vi "Config.vi"(8 "error in (no error)":errorcluster, 10 "Setting":variant, 11 "niPower in":refnum<class "NI DC Power.lvclass">) -> (0 "error out":errorcluster, 3 "niPower out":refnum<class "NI DC Power.lvclass">)   [LabVIEW 2025, in "Power Supply.lvlib" / "NI DC Power.lvclass"]
uses:
  NI DC Power.lvclass
  <instrlib>/niDCPower/nidcpower.llb/niDCPower Wait For Event - Event.ctl
  PS Channel/Power Supply Channel.lvclass
  NI DC Power.lvclass/NI DC Power.ctl
  <instrlib>/niDCPower/nidcpower.llb/niDCPower Output Function.ctl
  <instrlib>/niDCPower/nidcpower.llb/niDCPower Source Mode.ctl
  Users/Public/Documents/Sandia National Labs/TSS Plugin/Abstract Engine.lvlibp/Plugin/Abstract/Abstract Instrument/Channel.ctl
  PS Channel configuration/Power Supply Channel configuration.lvclass
  PS Channel configuration/Power Supply Channel configuration.lvclass/Power Supply Channel configuration.ctl
  PS Channel configuration/Read PS Channel.vi
  Users/Public/Documents/Sandia National Labs/TSS Plugin/CEF.lvlibp/Node/ReadChildren.vi
  Users/Public/Documents/Sandia National Labs/TSS Plugin/Abstract Engine.lvlibp/Plugin/Abstract/Channel configuration/Read Channel Setting.vi
  Users/Public/Documents/Sandia National Labs/TSS Plugin/CEF.lvlibp/Node/CEF_Node.lvclass
  Users/Public/Documents/Sandia National Labs/TSS Plugin/CEF.lvlibp/serializable configuration/CEF_serializable configuration.lvclass
  Users/Public/Documents/Sandia National Labs/TSS Plugin/Abstract Engine.lvlibp/Plugin/Abstract/Abstract Instrument/Abstract Instrument.lvclass
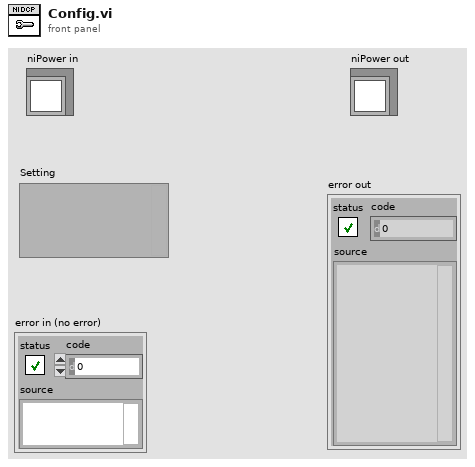
[diagram p1: front panel]
types:
  T1 = typedef "niDCPower Wait For Event - Event.ctl" = i32
  T2 = typedef "Abstract Engine.lvlibp/Abstract Instrument.lvclass/Channel.ctl" = cluster{"Alias":string, "DataType":enum16{"Anaolg Input", "Waveform"}, "Unit":enum16{"---", "V", "A", "Ohm", "Hz", "uF", "degC", "deg"}, "Upper limit":dbl, "Lower limit":dbl, "Measurement":variant}
  T3 = typedef "niDCPower Source Mode.ctl" = i32
  T4 = typedef "niDCPower Output Function.ctl" = i32
  T5 = typedef "Power Supply.lvlib/Power Supply Channel configuration.lvclass/PS Channel Setting.ctl" = cluster{"Driver":string, "Pin":string, "Test Voltage":string, "Voltage Low":dbl, "Voltage Norminal":dbl, "Voltage High":dbl, "PreTest Voltage":dbl, "PreTest Current":dbl, "Current Limit":dbl}
  T6 = typedef "Abstract Engine.lvlibp/Channel configuration.lvclass/Default Channel.ctl" = cluster{"Address":string, "SW Alias":string, "Enabled":bool, "Type":string, "Description":string}
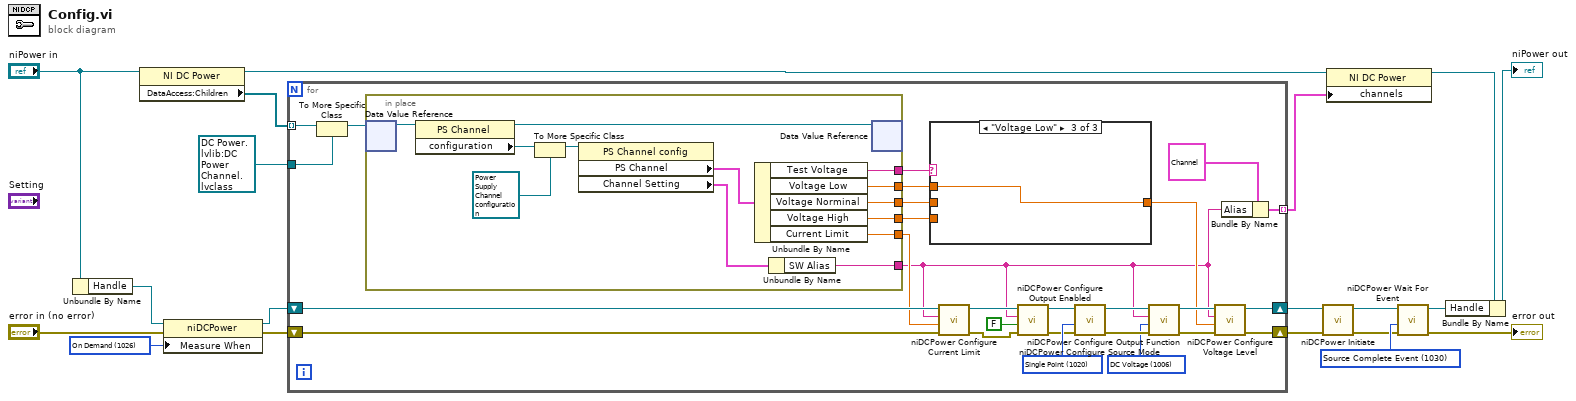
[diagram p0: block diagram]
diagram:
  w9 = 1026 items=["Automatically after Source Complete"=1025, "On Demand"=1026, "On Measure Trigger"=1027] ("Measurement:Advanced:Measure When")
  w17 = T1 1030 items=["Source Complete Event"=1030, "Measure Complete Event"=1031, "Sequence Iteration Complete Event"=1032, "Sequence Engine Done Event"=1033, "Pulse Complete Event"=1051, "Ready For Pulse Trigger Event"=1052] ("event")
  n1 = Unbundle By Name("niPower in") -> ("Handle"=w6:refnum<k15>)
  n2 = property class="NI DC Power"(reference="niPower in") -> (reference out=w12:refnum<class "NI DC Power.lvclass">, "DataAccess:Children"=w11:refnum<data-value>[])  [unwired: 1 in, 1 out]
  n3 = property class="niDCPower"(reference=w6, error in="error in (no error)", "Measure When"=w9) -> (reference out=w5:refnum<k15>, error out=w7:errorcluster)
  n4 = for {
    shift-right: [w27] -> w3
    shift-left: w5 -> [w26]
    shift-right: [w28] -> w4
    shift-left: w7 -> [w25]
    tunnel: w11 -> [w37] mode=indexing
    tunnel: refnum<data-value> refnum ("data value reference") -> [w35]
    tunnel: [w34] -> w1 mode=indexing
    w41 = T3 1020 items=["Single Point"=1020, "Sequence"=1021] ("source mode")
    w42 = T4 1006 items=["DC Voltage"=1006, "DC Current"=1007, "Pulse Voltage"=1049, "Pulse Current"=1050] ("output function")
    n5 = To More Specific Class(target class=w35, reference=w37) -> (specific class reference=w36:refnum<data-value>)  [unwired: 1 in, 1 out]
    n6 = in-place {
      in-place-border: [w47] -> w22
      in-place-border: [w57] -> w21
      in-place-border: [w51] -> w33
      in-place-border: [w50] -> w32
      in-place-border: [w49] -> w31
      in-place-border: [w48] -> w30
      # "Initialize the front panel controls when loaded"
      n7 = in-place-dvr #1(w36) -> (w59:refnum<class "Power Supply Channel.lvclass">)  [unwired: 1 out]
      n8 = property class="PS Channel"(reference=w59) -> (reference out=w58:refnum<class "Power Supply Channel.lvclass">, "configuration"=w56:refnum<class "CEF_serializable configuration.lvclass">)  [unwired: 1 in, 1 out]
      n9 = To More Specific Class(target class=refnum<class "Power Supply Channel configuration.lvclass"> refnum ("DC Power.lvlib:DCPower Channel configuration.lvclass"), reference=w56) -> (specific class reference=w55:refnum<class "Power Supply Channel configuration.lvclass">)  [unwired: 1 in, 1 out]
      n10 = property class="PS Channel config"(reference=w55) -> ("PS Channel"=w53:T5, "Channel Setting"=w52:T6)  [unwired: 1 in, 2 out]
      n11 = Unbundle By Name(w53) -> ("Test Voltage"=w51:string, "Voltage Low"=w50:dbl, "Voltage Norminal"=w49:dbl, "Voltage High"=w48:dbl, "Current Limit"=w47:dbl)
      n12 = Unbundle By Name(w52) -> ("SW Alias"=w57:string)
      n13 = in-place-dvr #1(w58) -> ()  [unwired: 2 out]
    }
    n14 = case shown="\"Voltage Low\"" w33 {
      tunnel: w32 -> [_ _ w62]
      tunnel: w31 -> [w60 _ _]
      tunnel: w30 -> [_ w61 _]
      tunnel: [w60 w61 w62] -> w29
      frame "Voltage Norminal", Default {
      }
      frame "Voltage High" {
      }
      frame "Voltage Low" {
      }
    }
    n15 = call <instrlib>:"niDCPower Configure Current Limit.vi"("error in (no error)"=w25, "current limit"=w22, "channel name"=w21, "instrument handle"=w26) -> ("error out"=w24:errorcluster, "instrument handle out"=w23:refnum<k15>)  [unwired: 6 in]
    n16 = call <instrlib>:"niDCPower Configure Output Enabled.vi"("error in (no error)"=w24, "output enabled"=FALSE, "channel name"=w21, "instrument handle"=w23) -> ("error out"=w39:errorcluster, "instrument handle out"=w40:refnum<k15>)  [unwired: 6 in]
    n17 = call <instrlib>:"niDCPower Configure Source Mode.vi"("error in (no error)"=w39, "source mode"=w41, "instrument handle"=w40) -> ("error out"=w46:errorcluster, "instrument handle out"=w45:refnum<k15>)  [unwired: 7 in]
    n18 = call <instrlib>:"niDCPower Configure Output Function.vi"("error in (no error)"=w46, "output function"=w42, "channel name"=w21, "instrument handle"=w45) -> ("error out"=w44:errorcluster, "instrument handle out"=w43:refnum<k15>)  [unwired: 6 in]
    n19 = call <instrlib>:"niDCPower Configure Voltage Level.vi"("error in (no error)"=w44, "voltage level"=w29, "channel name"=w21, "instrument handle"=w43) -> ("error out"=w28:errorcluster, "instrument handle out"=w27:refnum<k15>)  [unwired: 6 in]
    n20 = Bundle By Name(cluster=T2 {"Alias"="ch0", "DataType"=enum."Anaolg Input", "Unit"=enum."V", "Upper limit"=10.0, "Lower limit"=-10.0, "Measurement"=variant} ("Channel"), "Alias"=w21) -> (w34:T2)
  }
  n21 = call <instrlib>:"niDCPower Initiate.vi"("error in (no error)"=w4, "instrument handle"=w3) -> ("error out"=w15:errorcluster, "instrument handle out"=w16:refnum<k15>)  [unwired: 8 in]
  n22 = property class="NI DC Power"(reference=w12, "channels"=w1) -> (reference out=w2:refnum<class "NI DC Power.lvclass">)  [unwired: 1 in, 1 out]
  n23 = call <instrlib>:"niDCPower Wait For Event.vi"("error in (no error)"=w15, "event"=w17, "instrument handle"=w16) -> ("error out"=→"error out":errorcluster, "instrument handle out"=w14:refnum<k15>)  [unwired: 7 in]
  n24 = Bundle By Name(cluster=w2, "Handle"=w14) -> (→"niPower out":refnum<class "NI DC Power.lvclass">)
